vi "ResizePathtoPane.vi"(5 "Borders in Percent(T) or Pixels (F)":bool, 6 "Adjust":u16(ring) items=["Height", "Width", "Both"], 7 "Minimal":T1, 8 "error in (no error)":errorcluster, 9 "Borders":T2, 10 "Path":refnum<vi>, 11 "PentaPanesGUI in":refnum<class "PentaPanes.lvclass">) -> (0 "error out":errorcluster, 3 "PentaPanesGUI out":refnum<class "PentaPanes.lvclass">)   [LabVIEW 2022 SP3, in "PentaPanesLibrary.lvlib" / "PentaPanes.lvclass"]
uses:
  PentaPanes.lvclass
  BordersCluster.ctl
  <vilib>/Utility/miscctls.llb/LVBoundsTypeDef.ctl
  <vilib>/Utility/miscctls.llb/LVPositionTypeDef.ctl
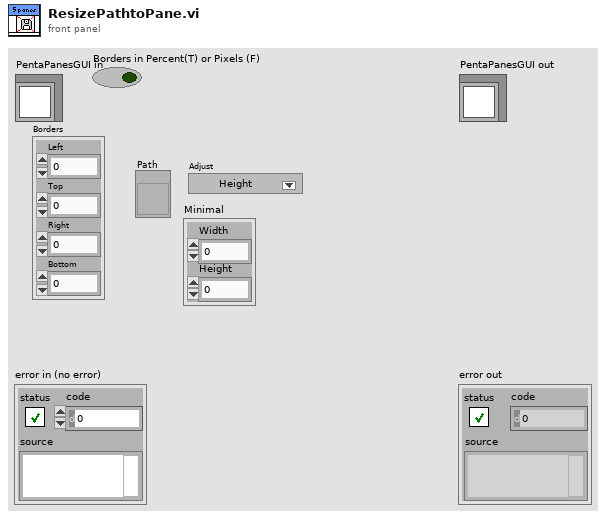
[diagram p1: front panel]
types:
  T1 = typedef "LVBoundsTypeDef.ctl" = cluster{"Width":i32, "Height":i32}
  T2 = typedef "PentaPanesLibrary.lvlib/PentaPanes.lvclass/BordersCluster.ctl" = cluster{"Left":i32, "Top":i32, "Right":i32, "Bottom":i32}
  T3 = typedef "LVPositionTypeDef.ctl" = cluster{"Left":i32, "Top":i32}
  T4 = typedef "LVBoundsTypeDef.ctl" = cluster{"Width":u32, "Height":u32}
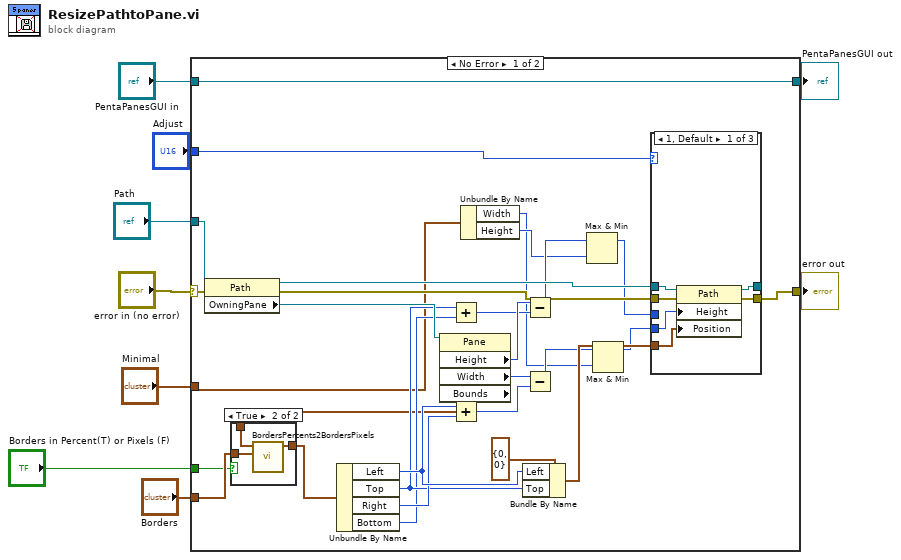
[diagram p0: block diagram]
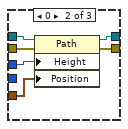
[diagram p3: hidden frame]
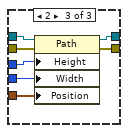
[diagram p4: hidden frame]
diagram:
  n1 = case shown="No Error" "error in (no error)" {
    selector: "error in (no error)" -> [w36 w63]
    tunnel: [w21 w63] -> w8
    tunnel: [w38 w62] -> w6
    tunnel: "PentaPanesGUI in" -> [w38 w62]
    tunnel: "Path" -> [w37 _]
    tunnel: "Borders" -> [w13 _]
    tunnel: "Adjust" -> [w33 _]
    tunnel: "Minimal" -> [w20 _]
    tunnel: "Borders in Percent(T) or Pixels (F)" -> [w10 _]
    frame No Error {
      n2 = property class="Path"(reference=w37, error in=w36) -> (reference out=w34:refnum<vi>, error out=w23:errorcluster, "OwningPane"=w35:refnum<vi>)
      n3 = property class="Pane"(reference=w35) -> ("Height"=w27:u32, "Width"=w25:u32, "Bounds"=w11:T4)  [unwired: 1 in, 2 out]
      n4 = case shown="True" w10 {
        tunnel: w11 -> [_ w42]
        tunnel: w13 -> [w39 w41]
        tunnel: [w39 w40] -> w12
        frame False {
        }
        frame True {
          n5 = call "BordersPercents2BordersPixels.vi"("Borders in"=w41, "Bounds"=w42) -> ("Borders out"=w40:T2)  [unwired: 9 in]
        }
      }
      n6 = Unbundle By Name(w12) -> ("Left"=w31:i32, "Top"=w29:i32, "Right"=w30:i32, "Bottom"=w28:i32)
      n7 = Add(x=w29, y=w28) -> (x+y=w26:i32)
      n8 = Add(x=w31, y=w30) -> (x+y=w24:i32)
      n9 = Unbundle By Name(w20) -> ("Width"=w14:i32, "Height"=w15:i32)
      n10 = Bundle By Name(cluster=T3 {"Left"=0, "Top"=0} ("Position"), "Left"=w31, "Top"=w29) -> (w22:T3)
      n11 = Subtract(x=w27, y=w26) -> (x-y=w19:u32)
      n12 = Subtract(x=w25, y=w24) -> (x-y=w18:u32)
      n13 = Max & Min(x=w19, y=w15) -> (max(x,y)=w16:u32)  [unwired: 1 out]
      n14 = Max & Min(x=w18, y=w14) -> (max(x,y)=w17:u32)  [unwired: 1 out]
      n15 = case shown="1, Default" w33 {
        tunnel: w34 -> [w48 w54 w61]
        tunnel: w16 -> [_ w53 w60]
        tunnel: w17 -> [w47 _ w59]
        tunnel: [w46 w52 w58] -> _
        tunnel: w23 -> [w45 w50 w56]
        tunnel: [w44 w51 w57] -> w21
        tunnel: w22 -> [w43 w49 w55]
        frame 1, Default {
          n16 = property class="Path"(reference=w48, error in=w45, "Height"=w47, "Position"=w43) -> (reference out=w46:refnum<vi>, error out=w44:errorcluster)
        }
        frame 0 {
          n17 = property class="Path"(reference=w54, error in=w50, "Height"=w53, "Position"=w49) -> (reference out=w52:refnum<vi>, error out=w51:errorcluster)
        }
        frame 2 {
          n18 = property class="Path"(reference=w61, error in=w56, "Height"=w60, "Width"=w59, "Position"=w55) -> (reference out=w58:refnum<vi>, error out=w57:errorcluster)
        }
      }
    }
    frame Error {
    }
  }
  "error out" <- w8
  "PentaPanesGUI out" <- w6
